vi "Test.vi"   [LabVIEW 2014]
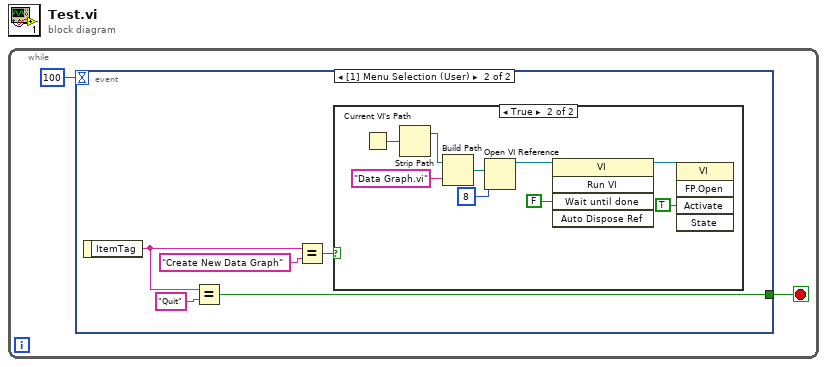
[diagram p0: block diagram]
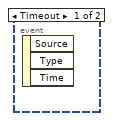
[diagram p2: hidden frame]
diagram:
  n1 = while {
    stop <- w1 stop-if-true
    n2 = event shown="[1] Menu Selection (User)" {
      selector: _ -> [_ _]
      dyn-events: _ -> [_ _]
      timeout: 100 -> [_ _]
      tunnel: [_ w6] -> w1
      event Timeout {
        n3 = event-data() -> ()  [unwired: 1 in, 3 out]
      }
      event Menu Selection (User) {
        n4 = event-data() -> ("ItemTag"=w4:string)  [unwired: 1 in]
        n5 = Equal?(x=w4, y="Quit") -> (x = y?=w6:bool)
        n6 = Equal?(x=w4, y="Create New Data Graph") -> (x = y?=w3:bool)
        n7 = case shown="True" w3 {
          frame False {
          }
          frame True {
            n8 = Current VI's Path() -> (path=w16:path)
            n9 = Strip Path(path=w16) -> (stripped path=w15:path)  [unwired: 1 out]
            n10 = Build Path(base path=w15, name or relative path="Data Graph.vi") -> (appended path=w13:path)
            n11 = Open VI Reference(vi path=w13, options=8) -> (vi reference=w12:refnum<vi>)  [unwired: 4 in, 1 out]
            n12 = invoke class="VI" method="Run VI"(reference=w12, "Wait until done"=FALSE ("Wait Until Done")) -> (reference out=w10:refnum<vi>)  [unwired: 3 in, 4 out]
            n13 = invoke class="VI" method="FP.Open"(reference=w10, "Activate"=TRUE ("Activate?")) -> ()  [unwired: 3 in, 5 out]
          }
        }
      }
    }
  }
